vi "specu1a 1.0.0 Read Calibration.vi"(3 "error in (no error)":errorcluster, 5 "Device Handle":i32) -> (0 "error out":errorcluster, 1 "Calibration":T1={"Offset"=0.0, "x"=1.0, "x^2"=2.0, "x^3"=3.0, "x^4"=4.0, "x^5"=5.0} {"x^5" format="%.2f"; "x^4" format="%.2f"; "x^3" format="%.2f"; "x^2" format="%.2f"; "x" format="%.2f"; "Offset" format="%.2f"}, 2 "Device Handle out":i32)   [LabVIEW 2010]
uses:
  Controls/specu1a 1.0.0 Calibration.ctl
  WINDOWS/SYSTEM32/DRIVERS/specu1a.dll
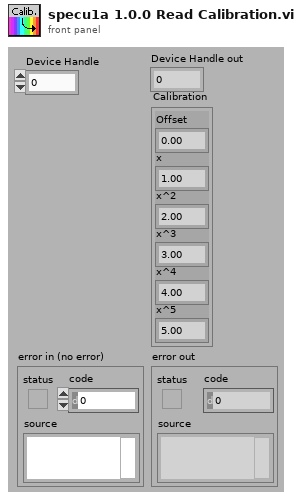
[diagram p1: front panel]
types:
  T1 = typedef "specu1a 1.0.0 Calibration.ctl" = cluster{"Offset":dbl, "x":dbl, "x^2":dbl, "x^3":dbl, "x^4":dbl, "x^5":dbl}
  T2 = typedef "specu1a 1.0.0 Error codes.ctl" = enum16{"INVALID_HANDLE_VALUE", "USBDEV_SUCCESS", "USBDEV_INVALID_HANDLE", "USBDEV_UNSUCCESS", "USBDEV_INVALID_VALUE", "USBDEV_CHECK_NORMAL", "USBDEV_CHECK_INVALID", "USBDEV_CHECK_REMOVE", "USBDEV_CHECK_OTHER", "USBDEV_RESET_ERROR", "USBDEV_BULKSIZE_ERROR", "USBDEV_BULK_READ_ERROR", "USBDEV_BULK_NOT_UPDATED", "USBDEV_TIME_OVER_ERROR", "USBDEV_TIME_UNDER_ERROR", "USBDEV_TIME_SET_ERROR", "USBDEV_SET_GAIN_ERROR", "USBDEV_GET_TEMP_ERROR", "USBDEV_SET_TRIGGER_ERROR", "USBDEV_RW_EEP_ADDR_ERROR", "USBDEV_RW_EEP_SIZE_ERROR", "USBDEV_RW_EEP_OVER_ERROR", "USBDEV_RW_EEP_ERROR", "UNITID_PRODUCTID_CONFLICT", "UNKNOWN_ERROR"}
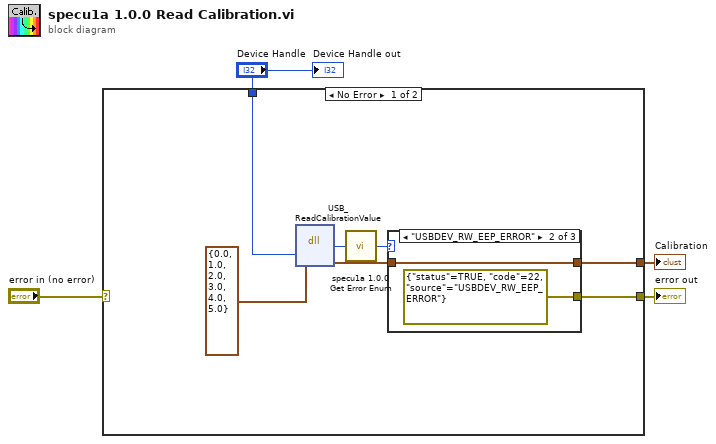
[diagram p0: block diagram]
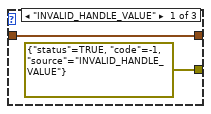
[diagram p2: hidden frame]
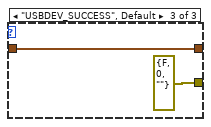
[diagram p3: hidden frame]
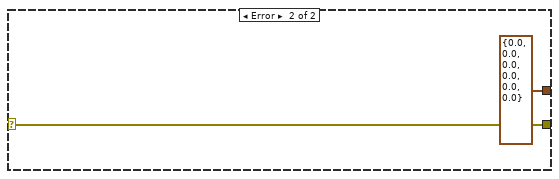
[diagram p4: hidden frame]
diagram:
  n1 = case shown="No Error" "error in (no error)" {
    selector: "error in (no error)" -> [_ w19]
    tunnel: [w10 w19] -> w3
    tunnel: [w9 T1 {"Offset"=0.0, "x"=0.0, "x^2"=0.0, "x^3"=0.0, "x^4"=0.0, "x^5"=0.0} ("Calibration")] -> w1
    tunnel: "Device Handle" -> [w8 _]
    frame No Error {
      n2 = dll-call lib="C:/WINDOWS/SYSTEM32/DRIVERS/specu1a.dll" fn="USB_ReadCalibrationValue" label="1.0.0 Read Calibration value"("Device Handle"=w8, "Calibration"=T1 {"Offset"=0.0, "x"=1.0, "x^2"=2.0, "x^3"=3.0, "x^4"=4.0, "x^5"=5.0}) -> (w6:u16, "Calibration"=w5:T1)  [unwired: 4 in, 2 out]
      n3 = call "specu1a 1.0.0 Get Error Enum.vi"("Error Code in"=w6) -> ("Specu1a 1.0.0 Error code out"=w11:T2)  [unwired: 4 in]
      n4 = case shown="\"USBDEV_RW_EEP_ERROR\"" w11 {
        tunnel: [w12 w14 w16] -> w9
        tunnel: [errorcluster {"status"=TRUE, "code"=-1, "source"="INVALID_HANDLE_VALUE"} ("error out") errorcluster {"status"=TRUE, "code"=22, "source"="USBDEV_RW_EEP_ERROR"} ("error out") errorcluster {"status"=FALSE, "code"=0, "source"=""} ("error out")] -> w10
        tunnel: w5 -> [w12 w14 w16]
        frame "INVALID_HANDLE_VALUE" {
        }
        frame "USBDEV_RW_EEP_ERROR" {
        }
        frame "USBDEV_SUCCESS", Default {
        }
      }
    }
    frame Error {
    }
  }
  "error out" <- w3
  "Calibration" <- w1
  "Device Handle out" <- "Device Handle"
